vi "Rad 2 PI-PI Vector.vi"(1 "vector in":dbl[](array[numeric])) -> (0 "vector out":dbl[](array[numeric]))   [LabVIEW 2014]
uses:
  <vilib>/imath/engines/lvmath2/RunTimeEngine/ArithmeticOperatorToken/NIMS_ArithmeticOperator_plus.vi
  <instcachedir>/0/NIMS_ArithmeticOperator_plus_48D6EAACA5D645B09F7EC9C016C2DEA8.lvgen/NIMS_ArithmeticOperator_plus_48D6EAACA5D645B09F7EC9C016C2DEA8_004.vi
  <vilib>/imath/engines/lvmath2/RunTimeEngine/BuiltInFunctions/rem/NIMS_rem_no checks.vi
  <instcachedir>/0/NIMS_rem_no checks_4BA74C9509D7485B8AB3E4C2ACC5A763.lvgen/NIMS_rem_no checks_4BA74C9509D7485B8AB3E4C2ACC5A763_001.vi
  <vilib>/imathl/engines/lvmath/Functions/Error Handling/Create Error.vi
  <vilib>/imath/engines/lvmath2/RunTimeEngine/BuiltInFunctions/abs/NIMS_abs(signed).vi
  <instcachedir>/0/NIMS_abs(signed)_C4FCB8E6058B49B797C7C8D53CA5F6EC.lvgen/NIMS_abs(signed)_C4FCB8E6058B49B797C7C8D53CA5F6EC_001.vi
  <vilib>/imath/engines/lvmath2/RunTimeEngine/ArithmeticOperatorToken/NIMS_ArithmeticOperator_minus.vi
  <instcachedir>/0/NIMS_ArithmeticOperator_minus_39C0593E74DA4138ACA2AB742906488D.lvgen/NIMS_ArithmeticOperator_minus_39C0593E74DA4138ACA2AB742906488D_003.vi
  <vilib>/imath/engines/lvmath2/RunTimeEngine/NodeEndStatement/NIMS_NodeEndStatement_Output.vi
  <instcachedir>/0/NIMS_NodeEndStatement_Output_53EC0D466D134D7ABD903AC30B43404B.lvgen/NIMS_NodeEndStatement_Output_53EC0D466D134D7ABD903AC30B43404B_005.vi
  <vilib>/imath/engines/lvmath2/RunTimeEngine/ErrorHandling/NIMS_Finalize Error.vi
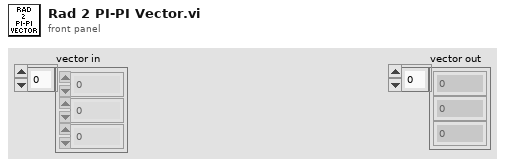
[diagram p1: front panel]
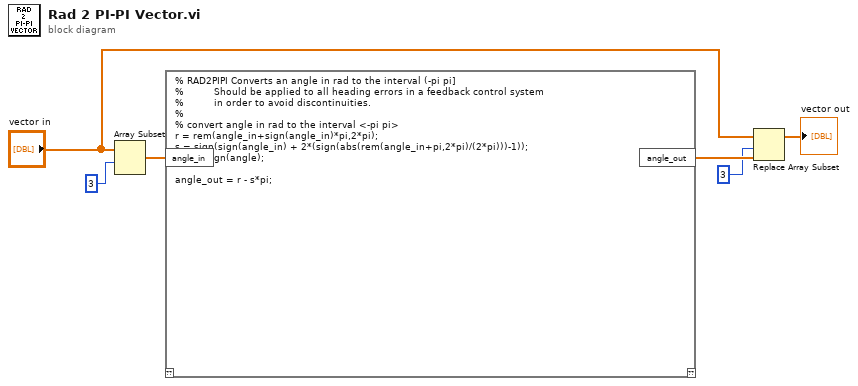
[diagram p0: block diagram]
diagram:
  n1 = Array Subset(array="vector in", index=3) -> (w6:dbl[])  [unwired: 1 in]
  n2 = mathscript code="% RAD2PIPI Converts an angle in rad to the interval (-pi pi]\n%          Should be applied to all heading errors in a feedback control system\n%          in order to avoid discontinuities.\n%\n% convert angle in rad to the interval <-pi pi> \nr = rem(angle_in+sign(angle_in)*pi,2*pi);\ns = sign(sign(angle_in) + 2*(sign(abs(rem(angle_in+pi,2*pi)/(2*pi)))-1));\n% s = sign(angle);\n\nangle_out = r - s*pi;"("angle_in"=w6) -> ("angle_out"=w5:dbl[])  [unwired: 1 in, 1 out]
  n3 = Replace Array Subset(array="vector in", new element=w5, index=3) -> (→"vector out":dbl[])
